vi "Offset by Point.vi"(8 "error in (no error)":errorcluster caption="错误输入（无错误）", 10 "Point Offset":refnum<class "Point.lvclass">, 11 "Point In":refnum<class "Point.lvclass">) -> (0 "error out":errorcluster caption="错误输出", 3 "Point Out":refnum<class "Point.lvclass">)   [LabVIEW 2011, in "Point.lvclass"]
uses:
  Point.lvclass
  Point.lvclass/Point.ctl
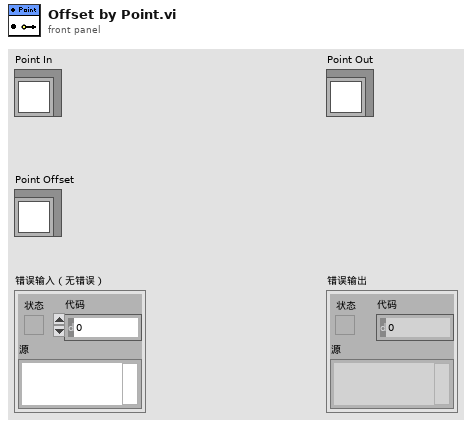
[diagram p1: front panel]
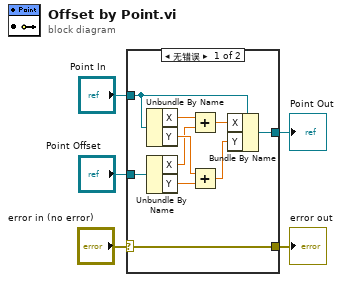
[diagram p0: block diagram]
diagram:
  n1 = case shown="无错误" "error in (no error)" {
    selector: "error in (no error)" -> [w15 w17]
    tunnel: [w15 w17] -> w4
    tunnel: "Point In" -> [w7 w16]
    tunnel: "Point Offset" -> [w8 _]
    tunnel: [w6 w16] -> w1
    frame No Error {
      n2 = Unbundle By Name(w7) -> ("X"=w9:dbl, "Y"=w11:dbl)
      n3 = Unbundle By Name(w8) -> ("X"=w10:dbl, "Y"=w12:dbl)
      n4 = Add(x=w9, y=w10) -> (x+y=w13:dbl)
      n5 = Add(x=w11, y=w12) -> (x+y=w14:dbl)
      n6 = Bundle By Name(cluster=w7, "X"=w13, "Y"=w14) -> (w6:refnum<class "Point.lvclass">)
    }
    frame Error {
    }
  }
  "Point Out" <- w1
  "error out" <- w4
